vi "SeCrTs-TC_Read_P3.vi"(8 "error in (no error)":errorcluster, 9 "Numeric":dbl, 10 "TC_Task":refnum<k21>, 11 "Data FIFO Ref":T1) -> (0 "error out":errorcluster, 2 "task out":refnum<k21>)   [LabVIEW 2022 SP3]
uses:
  RT Controls/SeCrTs-Data FIFO.ctl
  <vilib>/Platform/TimedLoop/XDataNode/timing_clust.ctl
  <vilib>/Platform/TimedLoop/XDataNode/nitl_modes.ctl
  <vilib>/Platform/TimedLoop/XDataNode/wakeup.ctl
  <vilib>/DAQmx/read.llb/DAQmx Read (Analog 1D Wfm NChan NSamp).vi
  <vilib>/DAQmx/miscellaneous.llb/DAQmx Fill In Error Info.vi
  <vilib>/platform/TimedLoop/XDataNode/XDataNode.xnode
  <vilib>/Platform/TimedLoop/XDataNode/XDNodeRunTimeDep.lvlib
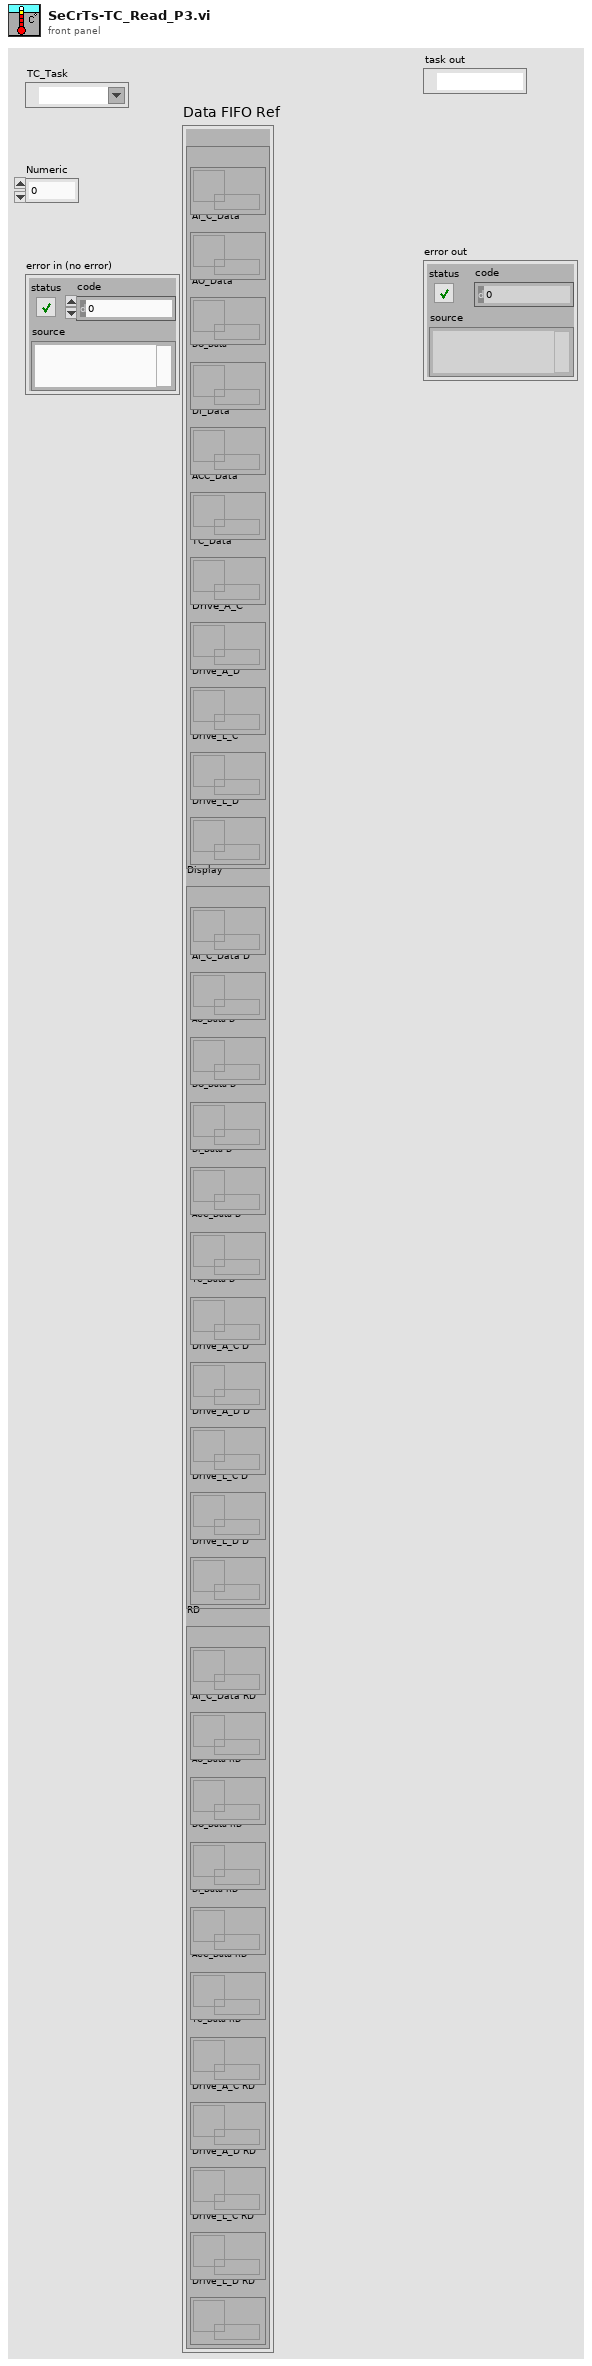
[diagram p1: front panel]
types:
  T1 = typedef "SeCrTs-Data FIFO.ctl" = cluster{"Control":cluster{"AI_V_Data":refnum<queue>, "AI_C_Data":refnum<queue>, "AO_Data":refnum<queue>, "DO_Data":refnum<queue>, "DI_Data":refnum<queue>, "ACC_Data":refnum<queue>, "TC_Data":refnum<queue>, "Drive_A_C":refnum<queue>, "Drive_A_D":refnum<queue>, "Drive_L_C":refnum<queue>, "Drive_L_D":refnum<queue>}, "Display":cluster{"AI_V_Data D":refnum<queue>, "AI_C_Data D":refnum<queue>, "AO_Data D":refnum<queue>, "DO_Data D":refnum<queue>, "DI_Data D":refnum<queue>, "ACC_Data D":refnum<queue>, "TC_Data D":refnum<queue>, "Drive_A_C D":refnum<queue>, "Drive_A_D D":refnum<queue>, "Drive_L_C D":refnum<queue>, "Drive_L_D D":refnum<queue>}, "RD":cluster{"AI_V_Data RD":refnum<queue>, "AI_C_Data RD":refnum<queue>, "AO_Data RD":refnum<queue>, "DO_Data RD":refnum<queue>, "DI_Data RD":refnum<queue>, "ACC_Data RD":refnum<queue>, "TC_Data RD":refnum<queue>, "Drive_A_C RD":refnum<queue>, "Drive_A_D RD":refnum<queue>, "Drive_L_C RD":refnum<queue>, "Drive_L_D RD":refnum<queue>}}
  T2 = typedef "XDNodeRunTimeDep.lvlib/timing_clust.ctl" = cluster{"Expected End [f-1]":u64, "Actual End [f-1]":u64, "Finished Late? [f-1]":bool, "Expected End [i-1]":u64, "Actual End [i-1]":u64, "Finished Late? [i-1]":bool, "Expected Start [i]":u64, "Actual Start [i]":u64, "Expected Start [f]":u64, "Actual Start [f]":u64, "Source Name":string, "Structure Name":string, "Period":i64, "Deadline":i64, "Offset":i64, "Start":i64, "Priority":i32, "Timeout":i32, "Mode":T3, "Wakeup Reason":T4, "Error":errorcluster, "Source Type":string, "Secondary Source Type":string, "Global End Time":u64, "Global Start Time":u64, "Frame Duration":u64, "Iteration Duration":u64, "Assigned CPU":i32, "I/O Scan Engine Mode":u32}
  T3 = typedef "XDNodeRunTimeDep.lvlib/nitl_modes.ctl" = enum32{"No Change", "Process missed periods, maintain original phase", "Discard missed periods, maintain original phase", "Process missed periods, ignore original phase", "Discard missed periods, ignore original phase"}
  T4 = typedef "XDNodeRunTimeDep.lvlib/wakeup.ctl" = enum32{"Normal", "Aborted", "Asynchronous wakeup", "Timing source error", "Timed loop error", "Timeout"}
  T5 = enum16{"AI C", "AI V", "AO", "DI", "DO", "TC", "ACC", "DR L", "DR A"}
  T6 = enum16{"Init", "Read 'All'", "Read 'n'", "Read '1'", "Write '1'", "Write 'n'", "Write 'All'"}
  T7 = cluster{"Start DAQ":bool, "Stop DAQ":bool, "RT Stop":bool, "RT Exit":bool, "Start Seq":bool}
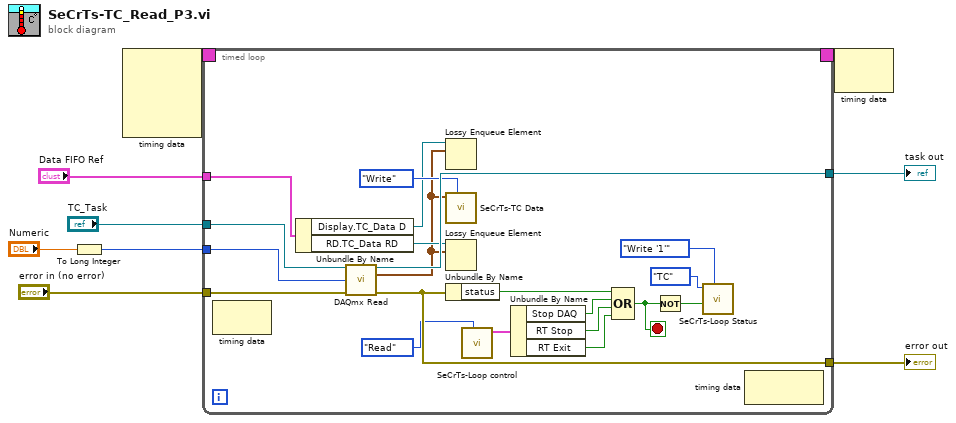
[diagram p0: block diagram]
diagram:
  n1 = To Long Integer(number="Numeric") -> (32bit integer=w3:i32)
  n2 = node-c288() -> (w2:T2)  [unwired: 4 in]
  n3 = timed-loop {
    tunnel: "error in (no error)" -> [w29]
    tunnel: "TC_Task" -> [w28]
    tunnel: w3 -> [w27]
    tunnel: [w26] -> w5
    tunnel: [w25] -> w9
    tunnel: "Data FIFO Ref" -> [w13]
    timing: w2 -> [_]
    timing-out: [_] -> w1
    stop <- w15 stop-if-true
    n4 = node-c288() -> ()  [unwired: 1 in, 1 out]
    n5 = Unbundle By Name(w13) -> ("Display.TC_Data D"=w12:refnum<queue>, "RD.TC_Data RD"=w11:refnum<queue>)
    n6 = call-poly <vilib>:"DAQmx Read.vi"("task/channels in"=w28, "number of samples per channel"=w27, "error in"=w29) -> ("task out"=w25:refnum<k21>, "data"=w10:waveform(dbl)[], "error out"=w26:errorcluster)  [unwired: 10 in]
    n7 = Lossy Enqueue Element(queue=w12, element=w10) -> ()  [unwired: 1 in, 4 out]
    n8 = call "SeCrTs-TC Data.vi"("Enum"=enum16{"Write", "Read"}."Write", "In_TC data"=w10) -> ()  [unwired: 9 in, 1 out]
    n9 = Lossy Enqueue Element(queue=w11, element=w10) -> ()  [unwired: 1 in, 4 out]
    n10 = Unbundle By Name(w26) -> ("status"=w24:bool)
    n11 = call "SeCrTs-Loop control.vi"("Action"=enum16{"Init", "Write", "Read"}."Read") -> ("Loop Control out"=w22:T7)  [unwired: 9 in, 1 out]
    n12 = Unbundle By Name(w22) -> ("Stop DAQ"=w21:bool, "RT Stop"=w20:bool, "RT Exit"=w19:bool)
    n13 = Compound Arithmetic op=OR(w24, w21, w20, w19) -> (w15:bool)
    n14 = Not(x=w15) -> (.not. x?=w16:bool)
    n15 = call "SeCrTs-Loop Status.vi"("Option"=T6."Write '1'", "Status"=w16, "Loop"=T5."TC") -> ()  [unwired: 6 in, 3 out]
    n16 = node-c288() -> ()  [unwired: 1 in, 1 out]
  }
  "task out" <- w9
  "error out" <- w5
  n17 = node-c288(w1) -> ()  [unwired: 1 out]
